vi "DPIO-Check Max SPL.vi"(0 "Max SPL":dbl, 5 "SPL Array":dbl[](array[numeric]), 7 "Channel":string, 11 "error in (no error)":errorcluster) -> (15 "error out":errorcluster)   [LabVIEW 2020]
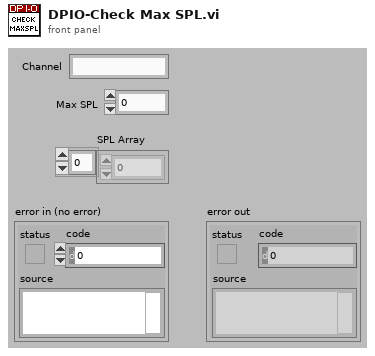
[diagram p1: front panel]
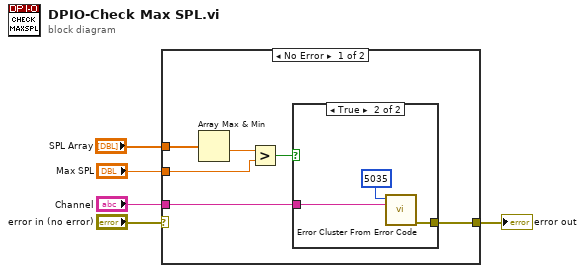
[diagram p0: block diagram]
diagram:
  n1 = case shown="No Error" "error in (no error)" {
    selector: "error in (no error)" -> [_ w15]
    tunnel: [w7 w15] -> w4
    tunnel: "SPL Array" -> [w11 _]
    tunnel: "Max SPL" -> [w9 _]
    tunnel: "Channel" -> [w6 _]
    frame No Error {
      n2 = Array Max & Min(array=w11) -> (min value=w10:dbl)  [unwired: 3 out]
      n3 = Greater?(x=w10, y=w9) -> (0:w8:bool)
      n4 = case shown="True" w8 {
        tunnel: [_ w14] -> w7
        tunnel: w6 -> [_ w12]
        frame False {
        }
        frame True {
          n5 = call <vilib>:"Error Cluster From Error Code.vi"("error message (\"\")"=w12, "error code (0)"=5035) -> ("error out"=w14:errorcluster)  [unwired: 7 in]
        }
      }
    }
    frame Error {
    }
  }
  "error out" <- w4
